vi "Base64 Encode.vi"(3 "Bytes":u8[](array[numeric])) -> (1 "Base64 sring out":string)   [LabVIEW 2020, in "wamplv.lvlib" / "Utils.lvclass"]
uses:
  Utils.lvclass
panel:
  # "Taken under MIT license, from\nhttps://forums.ni.com/t5/Example-Code/Fast-Base64-Encoder-Decoder-using-LabVIEW/ta-p/3503281"
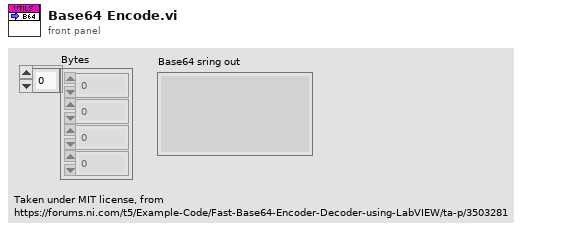
[diagram p1: front panel]
types:
  T1 = cluster{"Bytes[0]":u8, "Bytes[1]":u8, "Bytes[2]":u8}
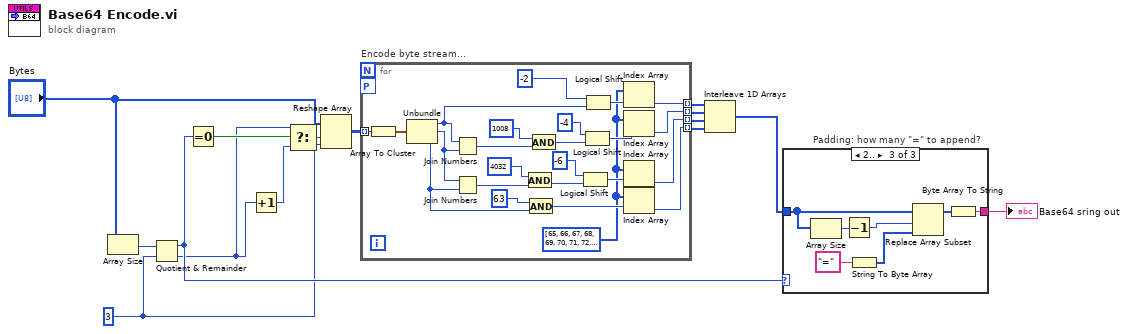
[diagram p0: block diagram]
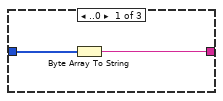
[diagram p2: hidden frame]
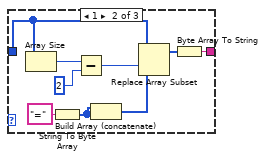
[diagram p3: hidden frame]
diagram:
  w4 = 3 ("y")
  n1 = Array Size(array="Bytes") -> (size(s)=w12:i32)
  n2 = Quotient & Remainder(x=w12, y=w4) -> (x-y*floor(x/y)=w13:i32, floor(x/y)=w6:i32)
  n3 = Equal To 0?(x=w13) -> (x = 0?=w14:bool)
  n4 = Increment(x=w6) -> (x+1=w7:i32)
  n5 = Select(t=w6, s=w14, f=w7) -> (s? t:f=w3:i32)
  n6 = Reshape Array("Bytes", w3, w4) -> (w2:u8[][])
  n7 = for "Encode byte stream..." {
    tunnel: [w18] -> w8 mode=indexing
    tunnel: [w19] -> w9 mode=indexing
    tunnel: [w20] -> w10 mode=indexing
    tunnel: [w21] -> w11 mode=indexing
    workers-P: _ -> [_]
    tunnel: w2 -> [w16] mode=indexing
    w17 = u8[] [65, 66, 67, 68, 69, 70, 71, 72, 73, 74, 75, 76, 77, 78, 79, 80, 81, 82, 83, 84, 85, 86, 87, 88, 89, 90, 97, 98, 99, 100, 101, 102, 103, 104, 105, 106, 107, 108, 109, 110, 111, 112, 113, 114, 115, 116, 117, 118, 119, 120, 121, 122, 48, 49, 50, 51, 52, 53, 54, 55, 56, 57, 43, 47] ("unsigned byte array")
    n8 = Array To Cluster(array=w16) -> (cluster=w39:T1)
    n9 = Unbundle(w39) -> ("Bytes[0]"=w28:u8, "Bytes[1]"=w33:u8, "Bytes[2]"=w27:u8)
    n10 = Join Numbers(hi=w28, lo=w33) -> ((hi.lo)=w37:u16)
    n11 = Join Numbers(hi=w33, lo=w27) -> ((hi.lo)=w32:u16)
    n12 = And(x=u16 4032, y=w32) -> (x .and. y?=w30:u16)
    n13 = And(x=u8 63, y=w27) -> (x .and. y?=w22:u8)
    n14 = And(x=u16 1008, y=w37) -> (x .and. y?=w35:u16)
    n15 = Logical Shift(y=i8 -6, x=w30) -> (x << y=w23:u16)
    n16 = Logical Shift(y=i8 -4, x=w35) -> (x << y=w24:u16)
    n17 = Logical Shift(y=i8 -2, x=w28) -> (x << y=w25:u8)
    n18 = Index Array(array=w17, index=w25) -> (element=w21:u8)
    n19 = Index Array(array=w17, index=w24) -> (element=w20:u8)
    n20 = Index Array(array=w17, index=w23) -> (element=w19:u8)
    n21 = Index Array(array=w17, index=w22) -> (element=w18:u8)
  }
  n22 = Interleave 1D Arrays(w11, w10, w9, w8) -> (w5:u8[])
  n23 = case "Padding: how many \"=\" to append?" shown="2.." w13 {
    tunnel: [w40 w47 w56] -> w15
    tunnel: w5 -> [w41 w45 w55]
    frame ..0 {
      n24 = Byte Array To String(unsigned byte array=w41) -> (string=w40:string)
    }
    frame 1 {
      n25 = Array Size(array=w45) -> (size(s)=w46:i32)
      n26 = String To Byte Array(string="=") -> (unsigned byte array=w43:u8[])
      n27 = Subtract(x=w46, y=2) -> (x-y=w49:i32)
      n28 = Build Array (concatenate)(w43, w43) -> (w42:u8[])
      n29 = Replace Array Subset(array=w45, new element=w42, index=w49) -> (w48:u8[])
      n30 = Byte Array To String(unsigned byte array=w48) -> (string=w47:string)
    }
    frame 2.. {
      n31 = Array Size(array=w55) -> (size(s)=w51:i32)
      n32 = Decrement(x=w51) -> (x-1=w52:i32)
      n33 = String To Byte Array(string="=") -> (unsigned byte array=w53:u8[])
      n34 = Replace Array Subset(array=w55, new element=w53, index=w52) -> (w57:u8[])
      n35 = Byte Array To String(unsigned byte array=w57) -> (string=w56:string)
    }
  }
  "Base64 sring out" <- w15
